vi "Do.vi"(8 "error in (no error)":errorcluster, 10 "Actor in":refnum<class "Actor.lvclass">, 11 "Turn mTEC on":refnum<class "Turn mTEC on.lvclass">) -> (0 "error out":errorcluster, 2 "Actor out":refnum<class "Actor.lvclass">)   [LabVIEW 2014, in "Controller.lvlib" / "Turn mTEC on.lvclass"]
doc: "(<B>Filename</B>: Actor Framework.lvlib:Message.lvclass:Do.vi)\n\nDefines what a message does when it is received by an actor. Generally, a message instructs an actor to invoke one of its methods. By default, this method does nothing. A child class must override it to define behavior. Create a child class by using the Actor Framework Message Maker dialog box."
uses:
  Turn mTEC on.lvclass
  <vilib>/ActorFramework/Actor/Actor.lvclass
  Turn mTEC on.lvclass/Turn mTEC on.ctl
  Controller.lvclass
  Controls/eMap.ctl
  <vilib>/ActorFramework/Message Enqueuer/Message Enqueuer.lvclass
  Controller.lvclass/Controller.ctl
  SuperActor/SuperActor.lvclass/SuperActor.ctl
  Devices/Meerstetter TEC/Meerstetter Output/Meerstetter output.lvclass
  Devices/Meerstetter TEC/Meerstetter Output/Meerstetter output.lvclass/Meerstetter output.ctl
  <vilib>/ActorFramework/Message Enqueuer/Message Enqueuer.lvclass/Message Enqueuer.ctl
  Devices/Meerstetter TEC/Meerstetter Output/Write Static On.vi
  Accessors/Read Enqueuer Map.vi
  SuperActor/Read Log Session.vi
  <vilib>/ActorFramework/Message Priority Queue/Priority Enqueue.vi
  <userlib>/_Session Fwk/Session - Root.lvclass
  reusable/Session APIs/Session Log/System Log.lvclass
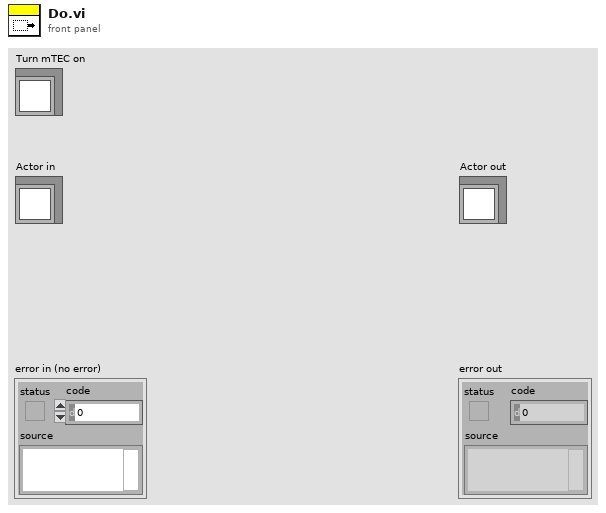
[diagram p1: front panel]
types:
  T1 = typedef "Controller.lvlib/Controller.lvclass/eMap.ctl" = cluster{"Enqueuer":refnum<class "Message Enqueuer.lvclass">, "Active":bool}
  T2 = typedef "Session - Root.lvclass/Session Handle.ctl" = refnum<data-value>
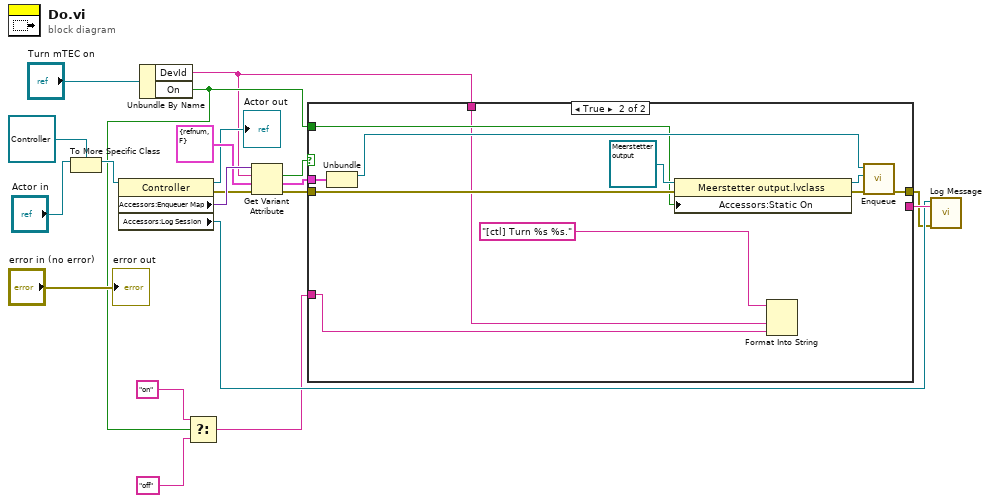
[diagram p0: block diagram]
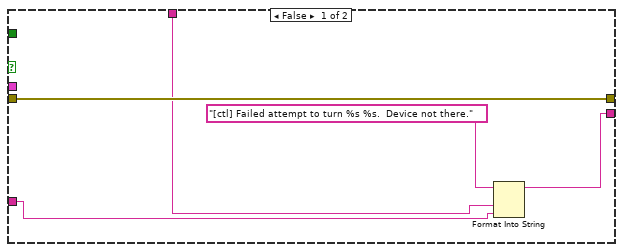
[diagram p2: hidden frame]
diagram:
  n1 = To More Specific Class(target class=refnum<class "Controller.lvclass"> refnum ("Controller:Controller"), reference="Actor in") -> (specific class reference=w19:refnum<class "Controller.lvclass">)  [unwired: 1 in, 1 out]
  n2 = property class="Controller"(reference=w19) -> (reference out=→"Actor out":refnum<class "Controller.lvclass">, error out=w16:errorcluster, "Accessors:Enqueuer Map"=w18:variant, "Accessors:Log Session"=w7:T2)  [unwired: 1 in]
  n3 = Unbundle By Name("Turn mTEC on") -> ("DevId"=w1:string, "On"=w5:bool)
  n4 = Select(t="on", s=w5, f="off") -> (s? t:f=w2:string)
  n5 = Get Variant Attribute(Variant=w18, name=w1, default value (empty Variant)=T1 {"Enqueuer"=refnum, "Active"=FALSE} ("eMap"), error in=w16) -> (found=w11:bool, value=w10:T1, error out=w9:errorcluster)  [unwired: 1 out]
  n6 = case shown="True" w11 {
    tunnel: w10 -> [_ w36]
    tunnel: w9 -> [w25 w33]
    tunnel: [w25 w31] -> w6
    tunnel: [w21 _] -> w8
    tunnel: w5 -> [_ w29]
    tunnel: w2 -> [w22 w26]
    tunnel: w1 -> [w23 w27]
    frame False {
      n7 = Format Into String(initial string="[ctl] Failed attempt to turn %s %s.  Device not there.", w23, w22) -> (resulting string=w21:string)  [unwired: 2 in, 1 out]
    }
    frame True {
      n8 = Unbundle(w36) -> ("Enqueuer"=w35:refnum<class "Message Enqueuer.lvclass">)  [unwired: 1 out]
      n9 = property class="Meerstetter output.lvclass"(reference=refnum<class "Meerstetter output.lvclass"> refnum ("Meerstetter Lib.lvlib:Meerstetter output.lvclass"), error in=w33, "Accessors:Static On"=w29) -> (reference out=w34:refnum<class "Meerstetter output.lvclass">, error out=w32:errorcluster)
      n10 = Format Into String(initial string="[ctl] Turn %s %s.", w27, w26) -> ()  [unwired: 2 in, 2 out]
      n11 = call <vilib>:"Enqueue.vi"("error in (no error)"=w32, "Message"=w34, "Message Enqueuer in"=w35) -> ("error out"=w31:errorcluster)  [unwired: 7 in, 1 out]
    }
  }
  n12 = call "Log Message.vi"("error in"=w6, "MSG In"=w8, "session in"=w7) -> ()  [unwired: 7 in, 2 out]
  "error out" <- "error in (no error)"
